vi "Preview Stack.vi"(8 "error in (no error)":errorcluster, 11 "Stack in":refnum<class "Stack.lvclass">) -> (0 "error out":errorcluster, 2 "Stack":dbl[](array[numeric]), 3 "Stack out":refnum<class "Stack.lvclass">)   [LabVIEW 2016, in "Stack.lvlib" / "Stack.lvclass"]
doc: "Returns the a preview of queue contents."
uses:
  Stack.lvclass
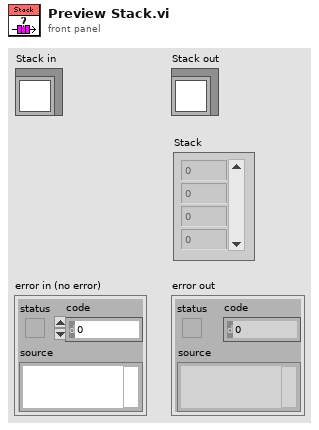
[diagram p1: front panel]
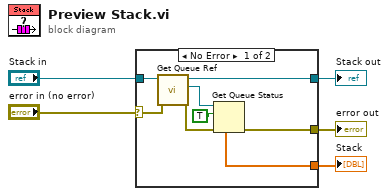
[diagram p0: block diagram]
diagram:
  n1 = case shown="No Error" "error in (no error)" {
    selector: "error in (no error)" -> [w9 w15]
    tunnel: [w8 w15] -> w4
    tunnel: [w12 w14] -> w2
    tunnel: "Stack in" -> [w13 w14]
    tunnel: [w6 _] -> w1
    frame No Error {
      n2 = call "Get Queue Ref.vi"("error in (no error)"=w9, "Stack in"=w13) -> ("error out"=w10:errorcluster, "queue out"=w11:refnum<queue>, "Stack out"=w12:refnum<class "Stack.lvclass">)  [unwired: 7 in]
      n3 = Get Queue Status(queue=w11, return elements? (F)=TRUE, error in (no error)=w10) -> (error out=w8:errorcluster, elements=w6:dbl[])  [unwired: 6 out]
    }
    frame Error {
    }
  }
  "error out" <- w4
  "Stack out" <- w2
  "Stack" <- w1
